vi "Send PLC Initialize Message.vi"(7 "Message Priority (Normal)":T2=enum."Normal", 8 "error in (no error)":errorcluster, 10 "Initialize Parameters":T1, 11 "Message Enqueuer":refnum<class "Message Enqueuer.lvclass">) -> (0 "error out":errorcluster, 3 "Message Enqueuer out":refnum<class "Message Enqueuer.lvclass">)   [LabVIEW 2022 SP3, in "Signal Acquisition.lvlib" / "PLC Initialize Message Msg.lvclass"]
doc: "This VI sends the message to an actor."
uses:
  PLC Initialize Message Msg.lvclass
  <vilib>/ActorFramework/Message Enqueuer/Message Enqueuer.lvclass
  <vilib>/ActorFramework/Message Enqueuer/Message Priority.ctl
  C:/Program Files/National Instruments/LabVIEW 2022/vi.lib/ActorFramework/Message/Message.lvclass
  PLC Initialize Message Msg.lvclass/PLC Initialize Message Msg.ctl
  <vilib>/ActorFramework/Message Enqueuer/Message Enqueuer.lvclass/Message Enqueuer.ctl
  <vilib>/ActorFramework/Message Priority Queue/Priority Enqueue.vi
  E:/image-harvest/Signal Acquisition/Signal Acquisition Messages/PLC Initialize Message Msg/PLC Initialize Message Msg.lvclass
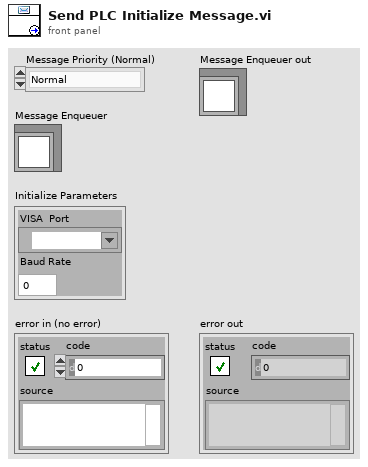
[diagram p1: front panel]
types:
  T1 = cluster{"VISA  Port":refnum<visa-resource-name>, "Baud Rate":u32}
  T2 = typedef "Actor Framework.lvlib/Message Enqueuer.lvclass/Message Priority.ctl" = enum16{"Low", "Normal", "High"}
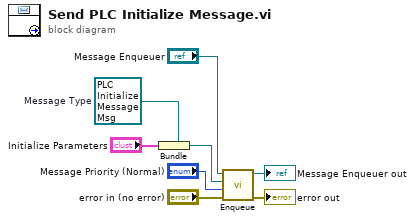
[diagram p0: block diagram]
diagram:
  w5 = refnum<class "PLC Initialize Message Msg.lvclass"> refnum  # Message Type
  n1 = Bundle(cluster=w5, "Initialize Parameters") -> (w4:refnum<class "PLC Initialize Message Msg.lvclass">)
  n2 = call <vilib>:"Enqueue.vi"("error in (no error)"="error in (no error)", "Message Priority (Normal)"="Message Priority (Normal)", "Message"=w4, "Message Enqueuer in"="Message Enqueuer") -> ("error out"=→"error out":errorcluster, "Message Enqueuer in"=→"Message Enqueuer out":refnum<class "Message Enqueuer.lvclass">)  [unwired: 6 in]
